vi "_Detect Peaks.vi"(4 "X Step":dbl=1.0, 5 "Masses":dbl[](array[numeric]), 6 "Minimum Height (0)":dbl, 7 "Minimum Width (4)":i32=4, 8 "Original Data":dbl[](array[numeric])) -> (1 "# of Peaks":i32, 2 "Locations":dbl[](array[numeric]), 3 "Peak List":T1[](array[typedef]))   [LabVIEW 2015]
uses:
  Type/_Peak Property.ctl
  <vilib>/Analysis/2dsp.llb/Derivative x(t).vi
  <vilib>/Analysis/NI_AALPro.lvlib
panel:
  in  "Peak":T1
  out "size":i32
  # "This algorithm has been optimized to process a data array of\n75,000 points with 6605 peaks in 100 mS."
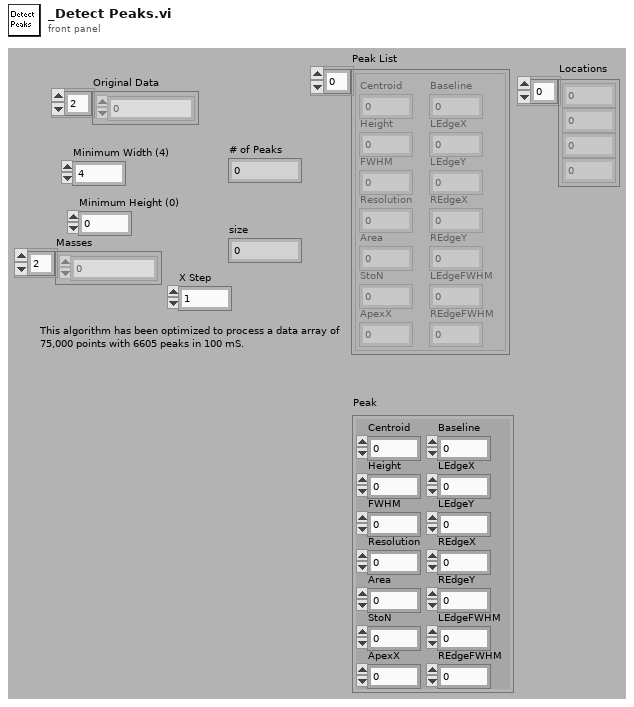
[diagram p1: front panel]
types:
  T1 = typedef "_Peak Property.ctl" = cluster{"Centroid":dbl, "Height":dbl, "FWHM":dbl, "Resolution":dbl, "Area":dbl, "StoN":dbl, "ApexX":dbl, "Baseline":dbl, "LEdgeX":dbl, "LEdgeY":dbl, "REdgeX":dbl, "REdgeY":dbl, "LEdgeFWHM":dbl, "REdgeFWHM":dbl}
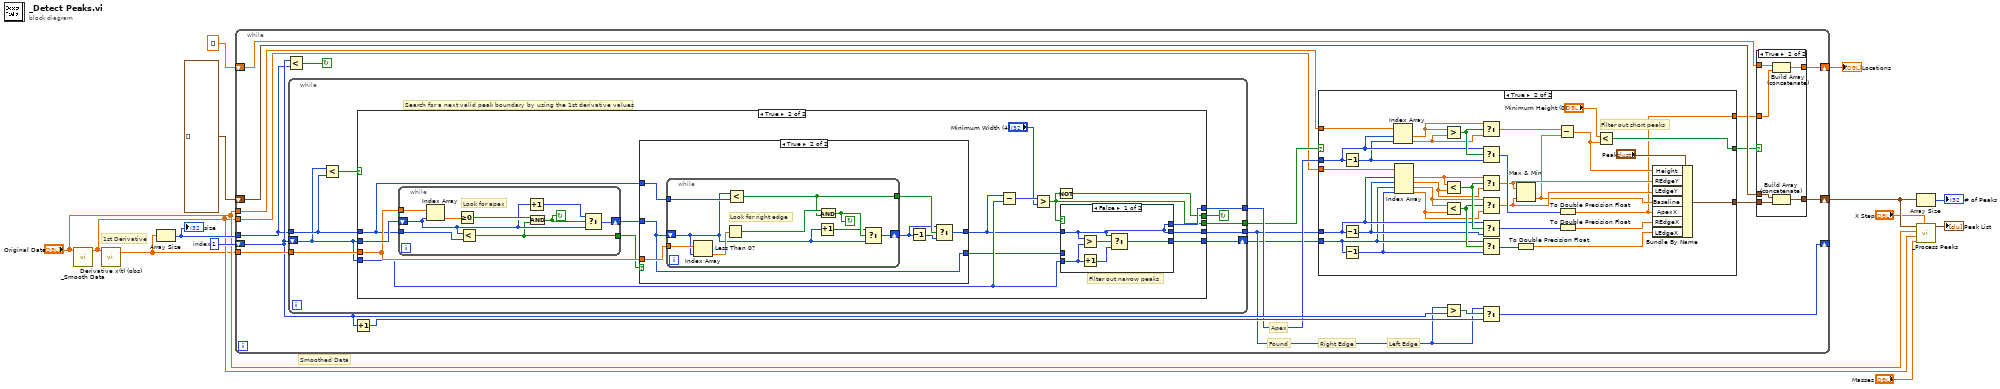
[diagram p0: block diagram]
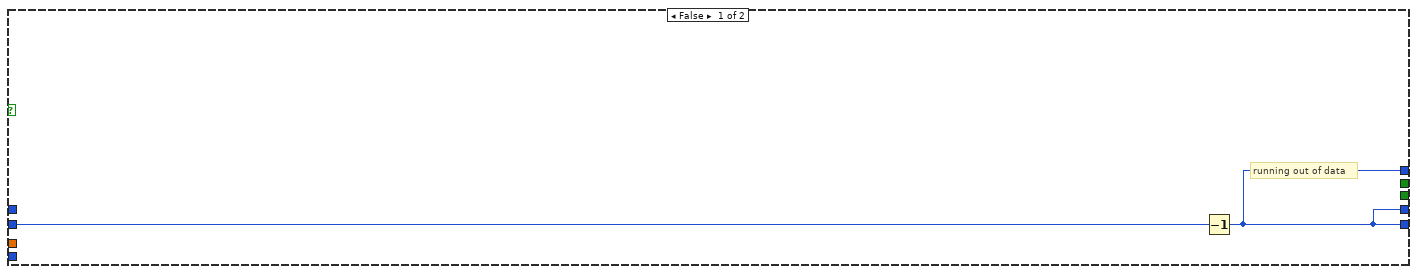
[diagram p3: hidden frame]
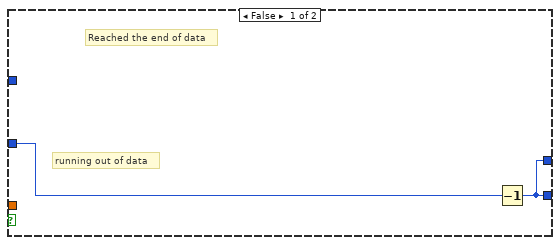
[diagram p4: hidden frame]
diagram:
  w12 = 1  # index
  # "Smoothed Data"
  # "1st Derivative"
  n1 = call "_Smooth Data.vi"("Data In"="Original Data") -> ("Data Out"=w6:dbl[])  [unwired: 6 out]
  n2 = call <vilib>:"Derivative x(t) (obs).vi"("X"=w6) -> ("dX/dt"=w5:dbl[])  [unwired: 3 in, 1 out]
  n3 = Array Size(array=w5) -> (size(s)=w13:i32)
  "size" <- w13
  n4 = while {
    tunnel: "Original Data" -> [w20]
    tunnel: w5 -> [w27]
    tunnel: w13 -> [w25]
    shift-right: [w28] -> _
    shift-left: w12 -> [w26]
    shift-right: [w32] -> w9
    shift-left: T1[] [] -> [w31]
    tunnel: w6 -> [w19]
    shift-right: [w14] -> w2
    shift-left: dbl[] [] ("Locations") -> [w16]
    stop <- w33 continue-if-true
    # "Found"
    # "Left Edge"
    # "Right Edge"
    # "Apex"
    n5 = Less?(x=w26, y=w25) -> (x < y?=w33:bool)
    n6 = while {
      tunnel: w27 -> [w75]
      tunnel: w25 -> [w68]
      shift-right: [w72] -> w22
      shift-left: w26 -> [w67]
      tunnel: [w71] -> w21
      tunnel: [w70] -> w24
      tunnel: [w69] -> w23
      stop <- w73 continue-if-true
      # "Search for a next valid peak boundary by using the 1st derivative values"
      n7 = Less?(x=w67, y=w68) -> (x < y?=w74:bool)
      n8 = case shown="True" w74 {
        tunnel: w75 -> [_ w85]
        tunnel: w67 -> [w77 w86]
        tunnel: [_ w89] -> w73
        tunnel: [w76 w87] -> w72
        tunnel: [_ w90] -> w71
        tunnel: [w76 w91] -> w70
        tunnel: [w76 w88] -> w69
        tunnel: w68 -> [_ w83]
        tunnel: w67 -> [_ w81]
        frame False {
          # "running out of data"
          n9 = Decrement(x=w77) -> (x-1=w76:i32)
        }
        frame True {
          # "Filter out narrow peaks"
          n10 = while {
            tunnel: w85 -> [w118]
            tunnel: w83 -> [w119]
            shift-right: [w112] -> w84
            shift-left: w86 -> [w113]
            tunnel: [w111] -> w82
            stop <- w115 continue-if-true
            # "Look for apex"
            n11 = Index Array(array=w118, index=w113) -> (element=w117:dbl)
            n12 = Greater Or Equal To 0?(x=w117) -> (x >= 0?=w116:bool)
            n13 = Less?(x=w113, y=w119) -> (x < y?=w111:bool)
            n14 = Increment(x=w113) -> (x+1=w114:i32)
            n15 = And(x=w116, y=w111) -> (x .and. y?=w115:bool)
            n16 = Select(t=w114, s=w115, f=w113) -> (s? t:f=w112:i32)
          }
          n17 = case shown="True" w82 {
            tunnel: w84 -> [w94 w95]
            tunnel: w83 -> [_ w101]
            tunnel: w85 -> [_ w100]
            tunnel: [w93 w99] -> w79
            tunnel: [w93 w95] -> w80
            frame False {
              # "running out of data"
              # "Reached the end of data"
              n18 = Decrement(x=w94) -> (x-1=w93:i32)
            }
            frame True {
              n19 = while {
                tunnel: w100 -> [w109]
                tunnel: w101 -> [w110]
                shift-right: [w104] -> w96
                shift-left: w95 -> [w103]
                tunnel: [w102] -> w98
                stop <- w106 continue-if-true
                # "Look for right edge"
                n20 = Index Array(array=w109, index=w103) -> (element=w108:dbl)
                n21 = Less Than 0?(x=w108) -> (x < 0?=w107:bool)
                n22 = Less?(x=w103, y=w110) -> (x < y?=w102:bool)
                n23 = Increment(x=w103) -> (x+1=w105:i32)
                n24 = And(x=w107, y=w102) -> (x .and. y?=w106:bool)
                n25 = Select(t=w105, s=w106, f=w103) -> (s? t:f=w104:i32)
              }
              n26 = Decrement(x=w96) -> (x-1=w97:i32)
              n27 = Select(t=w96, s=w98, f=w97) -> (s? t:f=w99:i32)
            }
          }
          n28 = Subtract(x=w79, y=w81) -> (x-y=w92:i32)
          n29 = Greater?(x=w92, y="Minimum Width (4)") -> (0:w90:bool)
          n30 = Not(x=w90) -> (.not. x?=w89:bool)
          n31 = case shown="False" w90 {
            tunnel: w80 -> [_ w127]
            tunnel: [w123 w127] -> w91
            tunnel: [w123 w126] -> w88
            tunnel: w79 -> [w123 w126]
            tunnel: w81 -> [w122 w125]
            tunnel: [w120 w125] -> w87
            frame False {
              n32 = Greater?(x=w123, y=w122) -> (0:w124:bool)
              n33 = Increment(x=w122) -> (x+1=w121:i32)
              n34 = Select(t=w123, s=w124, f=w121) -> (s? t:f=w120:i32)
            }
            frame True {
            }
          }
        }
      }
    }
    n35 = Increment(x=w26) -> (x+1=w29:i32)
    n36 = case shown="True" w21 {
      selector: w21 -> [w34 _]
      tunnel: w22 -> [_ w50]
      tunnel: w23 -> [_ w52]
      tunnel: w24 -> [_ w48]
      tunnel: [w34 w41] -> w17
      tunnel: [_ w40] -> w18
      tunnel: w20 -> [_ w38]
      tunnel: w19 -> [_ w37]
      tunnel: [_ w35] -> w15
      frame False {
      }
      frame True {
        # "Filter out short peaks"
        n37 = Decrement(x=w48) -> (x-1=w47:i32)
        n38 = Decrement(x=w52) -> (x-1=w51:i32)
        n39 = Decrement(x=w50) -> (x-1=w49:i32)
        n40 = Index Array(array=w38, index #1=w48, index #2=w47) -> (element #1=w54:dbl, element #2=w53:dbl)
        n41 = Index Array(array=w37, index #1=w52, index #2=w51, index #3=w50, index #4=w49) -> (element #1=w46:dbl, element #2=w45:dbl, element #3=w44:dbl, element #4=w43:dbl)
        n42 = Greater?(x=w54, y=w53) -> (0:w63:bool)
        n43 = Less?(x=w46, y=w45) -> (x < y?=w61:bool)
        n44 = Less?(x=w44, y=w43) -> (x < y?=w59:bool)
        n45 = Select(t=w54, s=w63, f=w53) -> (s? t:f=w64:dbl)
        n46 = Select(t=w48, s=w63, f=w47) -> (s? t:f=w62:i32)
        n47 = Select(t=w46, s=w61, f=w45) -> (s? t:f=w57:dbl)
        n48 = Select(t=w44, s=w59, f=w43) -> (s? t:f=w56:dbl)
        n49 = Select(t=w52, s=w61, f=w51) -> (s? t:f=w60:i32)
        n50 = Select(t=w50, s=w59, f=w49) -> (s? t:f=w58:i32)
        n51 = Max & Min(x=w57, y=w56) -> (min(x,y)=w55:dbl)  [unwired: 1 out]
        n52 = To Double Precision Float(number=w58) -> (double precision float=w65:dbl)
        n53 = Subtract(x=w64, y=w55) -> (x-y=w42:dbl)
        n54 = To Double Precision Float(number=w62) -> (double precision float=w35:dbl)
        n55 = To Double Precision Float(number=w60) -> (double precision float=w66:dbl)
        n56 = Less?(x="Minimum Height (0)", y=w42) -> (x < y?=w41:bool)
        n57 = Bundle By Name(cluster="Peak", "Height"=w42, "REdgeY"=w57, "LEdgeY"=w56, "Baseline"=w55, "ApexX"=w35, "REdgeX"=w66, "LEdgeX"=w65) -> (w40:T1)
      }
    }
    n58 = Greater?(x=w23, y=w26) -> (0:w30:bool)
    n59 = Select(t=w23, s=w30, f=w29) -> (s? t:f=w28:i32)
    n60 = case shown="True" w17 {
      tunnel: w18 -> [_ w135]
      tunnel: [w129 w134] -> w32
      tunnel: w31 -> [w129 w133]
      tunnel: w16 -> [w128 w131]
      tunnel: w15 -> [_ w132]
      tunnel: [w128 w130] -> w14
      frame False {
      }
      frame True {
        n61 = Build Array (concatenate)(w131, w132) -> (w130:dbl[])
        n62 = Build Array (concatenate)(w133, w135) -> (w134:T1[])
      }
    }
  }
  "Locations" <- w2
  n63 = Array Size(array=w9) -> (size(s)=→"# of Peaks":i32)
  n64 = call "_Process Peaks.vi"("X Step"="X Step", "Masses"="Masses", "Smoothed Data"=w6, "Original Data"="Original Data", "Peak List in"=w9) -> ("Peak List out"=→"Peak List":T1[])  [unwired: 3 out]
